vi "GetType.vi"(8 "error in (no error)":errorcluster, 11 "Create Arbitrary Sequence [SEQ] Msg":refnum<class "Create Arbitrary Sequence [SEQ] Msg.lvclass">) -> (0 "error out":errorcluster, 2 "Data Sample":variant, 3 "Create Arbitrary Sequence [SEQ] Msg":refnum<class "Create Arbitrary Sequence [SEQ] Msg.lvclass">)   [LabVIEW 2016, in "CS++Fgen.lvlib" / "Create Arbitrary Sequence [SEQ] Msg.lvclass"]
doc: "This VI delivers a sample of the data type format the message expects."
uses:
  Create Arbitrary Sequence [SEQ] Msg.lvclass
  Create Arbitrary Sequence [SEQ] Msg.lvclass/Create Arbitrary Sequence [SEQ] Msg.ctl
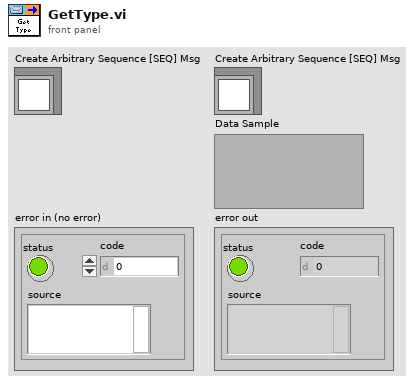
[diagram p1: front panel]
types:
  T1 = cluster{"loop counts array (empty)":i32[], "waveform handles array (empty)":i32[]}
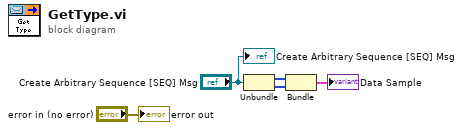
[diagram p0: block diagram]
diagram:
  n1 = Unbundle("Create Arbitrary Sequence [SEQ] Msg") -> (w2:i32[], w1:i32[])
  n2 = Bundle("loop counts array (empty)"=w2, "waveform handles array (empty)"=w1) -> (→"Data Sample":T1)  [unwired: 1 in]
  "error out" <- "error in (no error)"
  "Create Arbitrary Sequence [SEQ] Msg" <- "Create Arbitrary Sequence [SEQ] Msg"
